vi "LBCB Data.vi"() -> ()   [LabVIEW 2009]
uses:
  lib/Launcher/Launcher Actions.ctl
  lib/Launcher/NoPanelAppTypes.ctl
  lib/Data Access Objects/Metadata/DAO Actions.ctl
  lib/Data Access Objects/Application/Number Of LBCBs.ctl
  lib/Data Access Objects/Metadata/Persistant DAO Actions.ctl
  lib/Global Data/Transactions/Dataset Source.ctl
panel:
  out "DOF Labels4":string[](array[string])=["X1", "X2", "Y1", "Z1", "Z2", "Z3"]
  out "DOF Labels 3":string[](array[string])=["X1", "X2", "Y1", "Z1", "Z2", "Z3"]
  out "LBCB 1 Act Data":dbl[][](array[numeric]) caption="LBCB 1 Data"
  out "LBCB 2 Act Data":dbl[][](array[numeric]) caption="LBCB 2 Data"
  in  "Force Offset Tag":u16(ring)
  in  "Cartesian Type":bool caption="Coord"
  in  "Label1 3":string="Combined"
  in  "Label1 2":string="LBCB 2"
  in  "Label1":string="LBCB 1"
  out "Combined Data":dbl[][](array[numeric]) caption="LBCB 2 Data"
  out "DOF Labels3":string[](array[string])=["Dx", "Dy", "Dz", "Rx", "Ry", "Rz"]
  out "LBCB 1 Cart Data":dbl[][](array[numeric]) caption="LBCB 1 Data"
  out "LBCB 2 Cart Data":dbl[][](array[numeric]) caption="LBCB 2 Data"
  out "DOF Labels 2":string[](array[string])=["Dx", "Dy", "Dz", "Rx", "Ry", "Rz"]
  out "DOF Labels":string[](array[string])=["Dx", "Dy", "Dz", "Rx", "Ry", "Rz"]
  in  "Ok":bool
  # "Actuator"
  # "Cartesian"
  # "Forces"
  # "Forces"
  # "Displacements"
  # "Displacements"
  # "Commands"
  # "Commands"
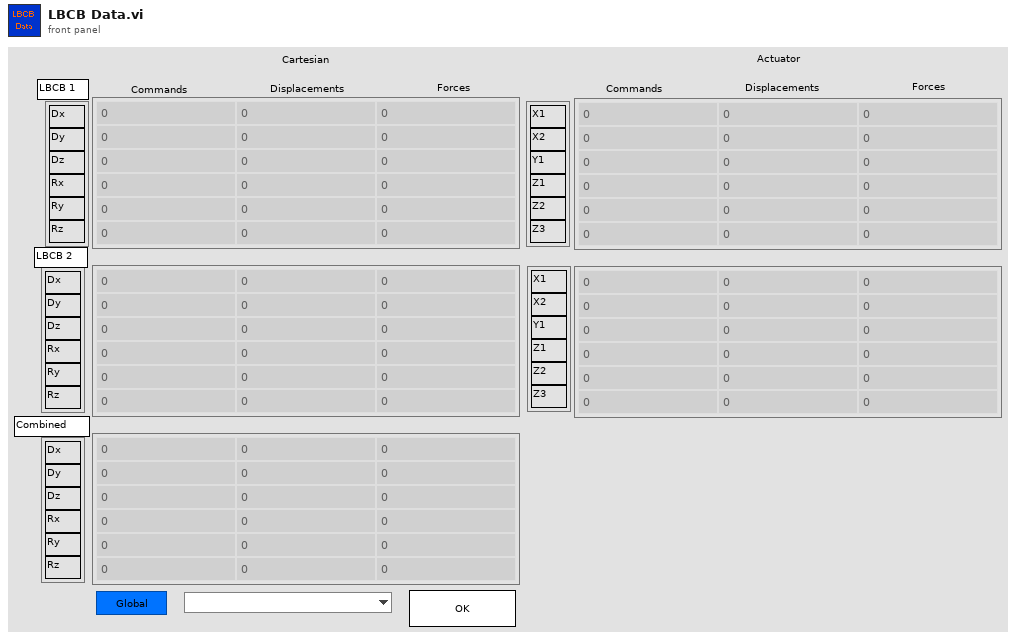
[diagram p1: front panel]
types:
  T1 = typedef "NoPanelAppTypes.ctl" = enum16{"NTCP Socket", "Data Archiving", "DAQ Link", "Control Loops", "Cmd Disp Diffs", "LBCB Cart Data", "Limits", "Mixed Mode Widget", "Offsets"}
  T2 = typedef "Launcher Actions.ctl" = enum16{"Launch", "Stop All", "Stop", "Kill", "Running?", "Init"}
  T3 = typedef "DAO Actions.ctl" = enum16{"Init", "Get", "Set"}
  T4 = typedef "Number Of LBCBs.ctl" = enum16{"1", "2"}
  T5 = typedef "Persistant DAO Actions.ctl" = enum16{"Init", "Get", "Set", "Load", "Save"}
  T6 = typedef "Dataset Source.ctl" = enum16{"LBCB 1", "LBCB 2", "Combined", "External Sensors"}
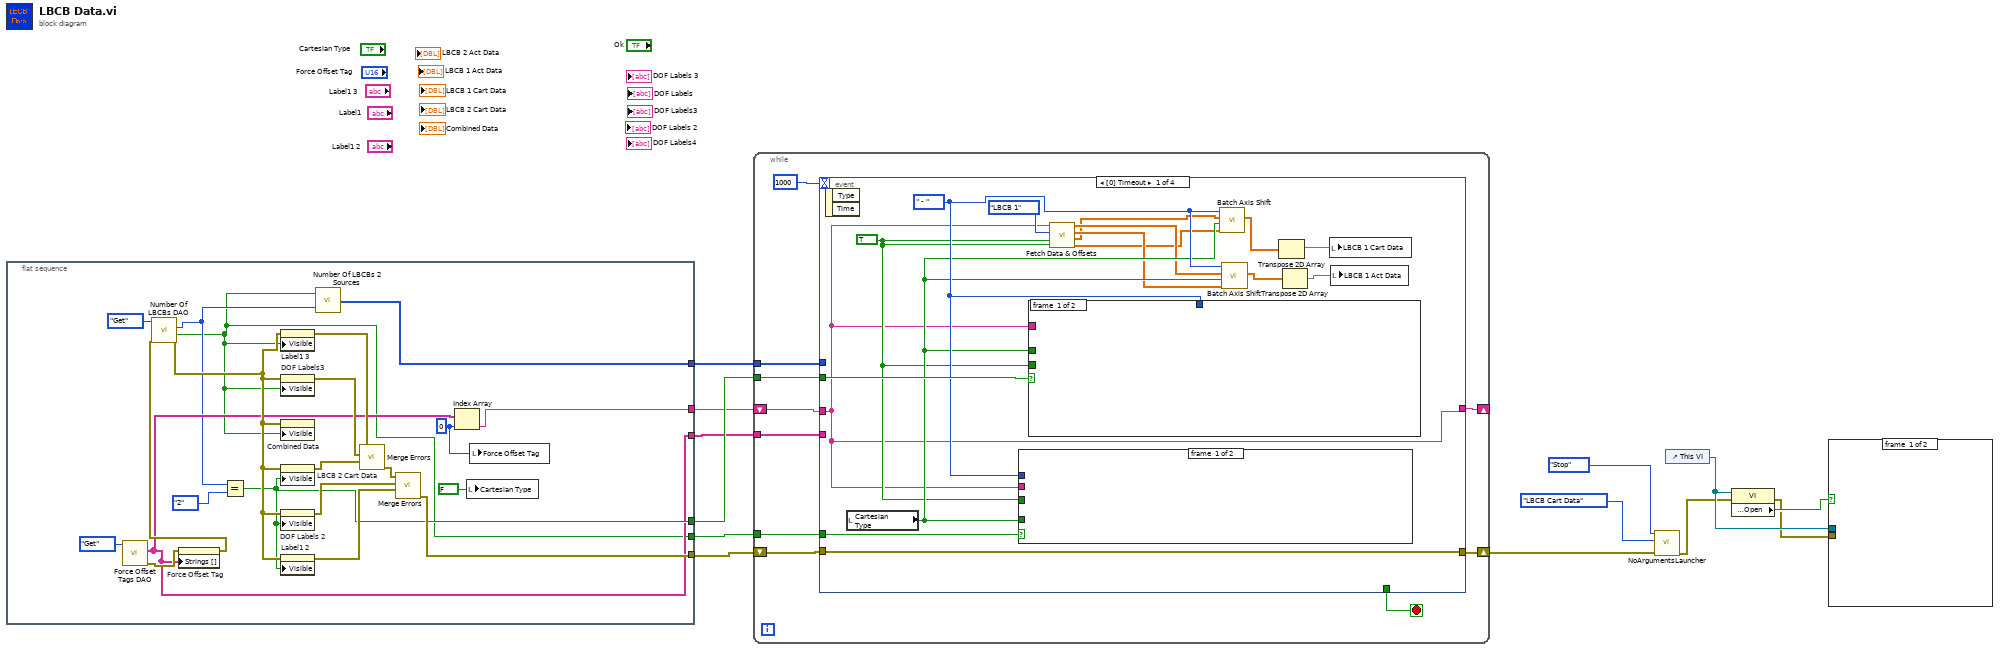
[diagram p0: block diagram]
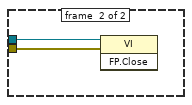
[diagram p2: hidden frame]
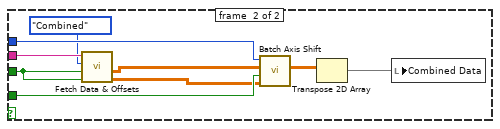
[diagram p3: hidden frame]
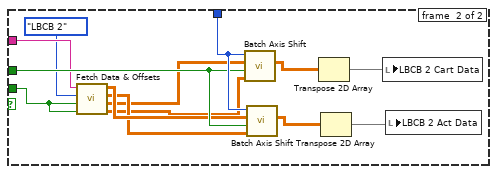
[diagram p4: hidden frame]
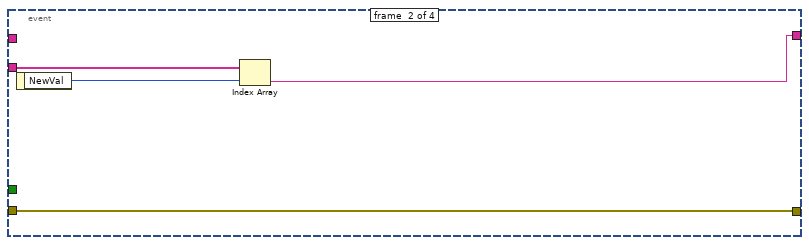
[diagram p5: hidden frame]
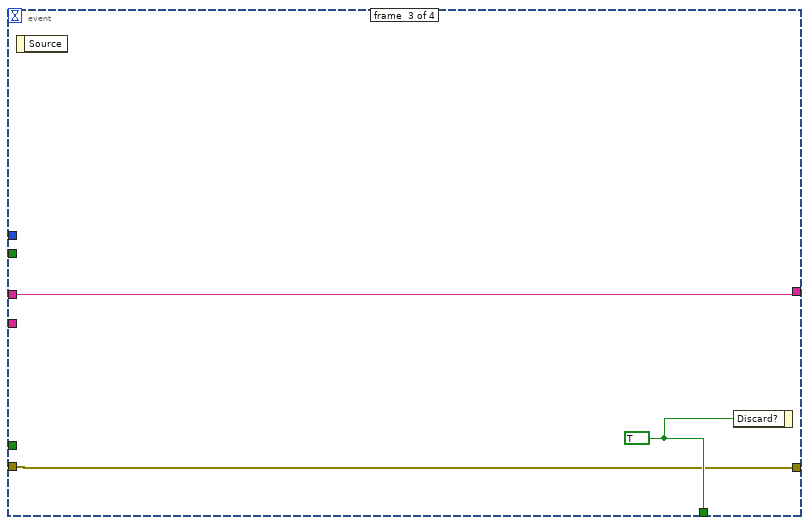
[diagram p6: hidden frame]
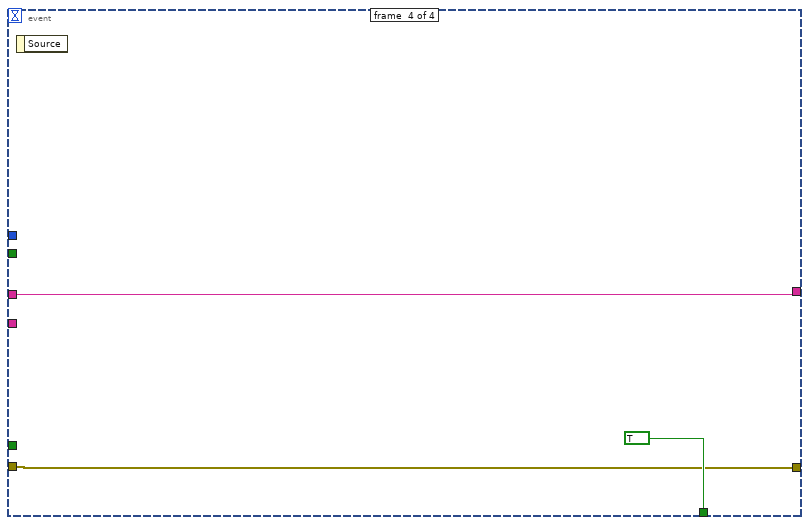
[diagram p7: hidden frame]
diagram:
  n1 = flat-sequence {
    tunnel: [w34] -> w10
    tunnel: [w16] -> w9
    tunnel: [w19] -> w8
    tunnel: [w18] -> w7
    tunnel: [w15] -> w2
    tunnel: [w14] -> w1
    frame #0 {
      w21 = 0 ("index")
      n2 = call "Force Offset Tags DAO.vi"("DAO Actions"=DAO_Actions."Get") -> ("error out"=w23:errorcluster, "Force Tags"=w18:string[])  [unwired: 9 in]
      n3 = property on="Force Offset Tag" class="Ring (strict)"(error in=w23, "Strings []"=w18) -> (error out=w22:errorcluster)  [unwired: 1 in, 1 out]
      n4 = call "Number Of LBCBs DAO.vi"("error in (no error)"=w22, "Actions"=Persistant_DAO_Actions."Get") -> ("error out"=w31:errorcluster, "Rigid Connection Out"=w16:bool, "Number of\nLBCBs Out"=w17:T4)  [unwired: 6 in, 1 out]
      n5 = Equal?(x=w17, y=Number_Of_LBCBs."2") -> (x = y?=w19:bool)
      n6 = property on="Label1 3" class="Str"(error in=w31, "Visible"=w16) -> (error out=w30:errorcluster)  [unwired: 1 in, 1 out]
      n7 = property on="DOF Labels3" class="Arr (strict)"(error in=w31, "Visible"=w16) -> (error out=w29:errorcluster)  [unwired: 1 in, 1 out]
      n8 = property on="Combined Data" class="Arr (strict)"(error in=w31, "Visible"=w16) -> ()  [unwired: 1 in, 2 out]
      n9 = property on="LBCB 2 Cart Data" class="Arr (strict)"(error in=w31, "Visible"=w19) -> (error out=w28:errorcluster)  [unwired: 1 in, 1 out]
      n10 = property on="DOF Labels 2" class="Arr (strict)"(error in=w31, "Visible"=w19) -> (error out=w26:errorcluster)  [unwired: 1 in, 1 out]
      n11 = property on="Label1 2" class="Str"(error in=w31, "Visible"=w19) -> (error out=w25:errorcluster)  [unwired: 1 in, 1 out]
      n12 = call "Number Of LBCBs 2 Sources.vi"("Number of LBCBs"=w17, "Combined LBCBs"=w16) -> ("Sources"=w14:T6[])
      n13 = call <vilib>:"Merge Errors.vi"("error in 3 (no error)"=w28, "error in 2 (no error)"=w29, "error in 1 (no error)"=w30) -> ("error out"=w27:errorcluster)  [unwired: 4 in]
      n14 = call <vilib>:"Merge Errors.vi"("error in 3 (no error)"=w25, "error in 2 (no error)"=w26, "error in 1 (no error)"=w27) -> ("error out"=w34:errorcluster)  [unwired: 4 in]
      n15 = Index Array(array=w18, index=w21) -> (element=w15:string)
      n16 = local write "Cartesian Type"(FALSE ("Cartesian Type")) -> ()
      n17 = local write "Force Offset Tag"(w21) -> ()
    }
  }
  n18 = while {
    shift-right: [w41] -> w11
    shift-left: w10 -> [w42]
    tunnel: w9 -> [w40]
    tunnel: w8 -> [w39]
    tunnel: w7 -> [w38]
    shift-right: [w35] -> _
    shift-left: w2 -> [w37]
    tunnel: w1 -> [w36]
    stop <- w43 stop-if-true
    n19 = event shown="[0] Timeout" {
      selector: _ -> [_ _ _ _]
      dyn-events: _ -> [_ _ _ _]
      timeout: 1000 -> [_ _ _ _]
      tunnel: [_ _ w89 TRUE] -> w43
      tunnel: w42 -> [w46 w84 w88 w91]
      tunnel: [w46 w84 w88 w91] -> w41
      tunnel: w40 -> [w58 _ _ _]
      tunnel: w39 -> [w57 _ _ _]
      tunnel: w38 -> [_ w86 _ _]
      tunnel: w37 -> [w47 _ w87 w90]
      tunnel: w36 -> [_ _ _ _]
      tunnel: [w47 w83 w87 w90] -> w35
      event #0 {
        w48 = TRUE ("Include Command")
        w55 = enum16{" +", " - "}." - " ("Direction")
        n20 = event-data() -> ()  [unwired: 3 out]
        n21 = local read "Cartesian Type"() -> (w54:bool)
        n22 = case shown="True" w58 {
          tunnel: w55 -> [_ w67]
          tunnel: w54 -> [_ w66]
          tunnel: w47 -> [_ w65]
          tunnel: w48 -> [_ w64]
          frame #0 {
          }
          frame #1 {
            n23 = call "Fetch Data & Offsets.vi"("Include Command"=w64, "Include Reading"=w64, "Source"=Dataset_Source."Combined", "Force Tag"=w65) -> ("Cartesian Offsets"=w61:dbl[][], "Cartesian Data"=w62:dbl[][])  [unwired: 2 out]
            n24 = call "Batch Axis Shift.vi"("Offsets In"=w61, "Coordinate Switch"=w66, "Data In"=w62, "Direction"=w67) -> ("Data Out"=w68:dbl[][])  [unwired: 7 in]
            n25 = Transpose 2D Array(2D array=w68) -> (transposed array=w69:dbl[][])
            n26 = local write "Combined Data"(w69) -> ()
          }
        }
        n27 = case shown="True" w57 {
          tunnel: w55 -> [_ w79]
          tunnel: w54 -> [_ w78]
          tunnel: w47 -> [_ w76]
          tunnel: w48 -> [_ w75]
          frame #0 {
          }
          frame #1 {
            n28 = call "Fetch Data & Offsets.vi"("Include Command"=w75, "Include Reading"=w75, "Source"=Dataset_Source."LBCB 2", "Force Tag"=w76) -> ("Cartesian Offsets"=w70:dbl[][], "Cartesian Data"=w71:dbl[][], "Actuator Offsets"=w72:dbl[][], "Actuator Data"=w73:dbl[][])
            n29 = call "Batch Axis Shift.vi"("Offsets In"=w70, "Coordinate Switch"=w78, "Data In"=w71, "Direction"=w79) -> ("Data Out"=w81:dbl[][])  [unwired: 7 in]
            n30 = call "Batch Axis Shift.vi"("Offsets In"=w72, "Coordinate Switch"=w78, "Data In"=w73, "Direction"=w79) -> ("Data Out"=w80:dbl[][])  [unwired: 7 in]
            n31 = Transpose 2D Array(2D array=w81) -> (transposed array=w82:dbl[][])
            n32 = Transpose 2D Array(2D array=w80) -> (transposed array=w77:dbl[][])
            n33 = local write "LBCB 2 Cart Data"(w82) -> ()
            n34 = local write "LBCB 2 Act Data"(w77) -> ()
          }
        }
        n35 = call "Fetch Data & Offsets.vi"("Include Command"=w48, "Include Reading"=w48, "Source"=Dataset_Source."LBCB 1", "Force Tag"=w47) -> ("Cartesian Offsets"=w50:dbl[][], "Cartesian Data"=w51:dbl[][], "Actuator Offsets"=w52:dbl[][], "Actuator Data"=w53:dbl[][])
        n36 = call "Batch Axis Shift.vi"("Offsets In"=w50, "Coordinate Switch"=w54, "Data In"=w51, "Direction"=w55) -> ("Data Out"=w59:dbl[][])  [unwired: 7 in]
        n37 = call "Batch Axis Shift.vi"("Offsets In"=w52, "Coordinate Switch"=w54, "Data In"=w53, "Direction"=w55) -> ("Data Out"=w56:dbl[][])  [unwired: 7 in]
        n38 = Transpose 2D Array(2D array=w59) -> (transposed array=w60:dbl[][])
        n39 = Transpose 2D Array(2D array=w56) -> (transposed array=w45:dbl[][])
        n40 = local write "LBCB 1 Cart Data"(w60) -> ()
        n41 = local write "LBCB 1 Act Data"(w45) -> ()
      }
      event #1 {
        n42 = event-data() -> ("NewVal"=w85:u16)  [unwired: 1 out]
        n43 = Index Array(array=w86, index=w85) -> (element=w83:string)
      }
      event #2 {
        w89 = TRUE
        n44 = event-data() -> ()  [unwired: 2 out]
        n45 = event-data("Discard?"=w89) -> ()  [unwired: 1 in, 1 out]
      }
      event #3 {
        n46 = event-data() -> ()  [unwired: 2 out]
      }
    }
  }
  n47 = call "NoArgumentsLauncher.vi"("error in (no error)"=w11, "Application"=NoPanelAppTypes."LBCB Cart Data", "Application Launcher Actions"=Launcher_Actions."Stop") -> ("error out"=w4:errorcluster)  [unwired: 8 out]
  n48 = control-ref of="This VI"() -> (w6:refnum<vi>)
  n49 = property class="VI"(reference=w6, error in=w4) -> (error out=w3:errorcluster, "Front Panel.Open"=w5:bool)  [unwired: 1 out]
  n50 = case shown="True" w5 {
    tunnel: w3 -> [_ w94]
    tunnel: w6 -> [_ w93]
    frame #0 {
    }
    frame #1 {
      n51 = invoke class="VI" method="FP.Close"(reference=w93, error in=w94) -> ()  [unwired: 1 in, 3 out]
    }
  }
